vi "Test Beep.vi"() -> ()   [LabVIEW 2016, in "CS++BeepActor.lvlib"]
doc: "Test Beep.vi"
uses:
  CS++BeepActor.lvlib
  Beep.lvclass
panel:
  in  "Duration":dbl[unit]=0.1
  in  "Frequency (440)":dbl[unit]=440.0
  in  "Use System Alert?":bool
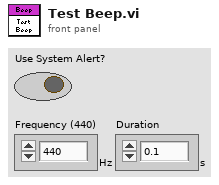
[diagram p1: front panel]
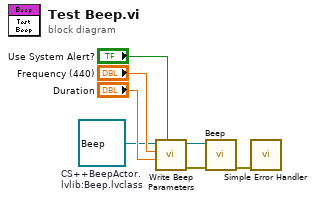
[diagram p0: block diagram]
diagram:
  w1 = refnum<class "Beep.lvclass"> refnum  # CS++BeepActor.lvlib:Beep.lvclass
  n1 = call "Write Beep Parameters.vi"("Use System Alert?"="Use System Alert?", "Duration"="Duration", "Frequency (440)"="Frequency (440)", "Beep in"=w1) -> ("error out"=w2:errorcluster, "Beep out"=w3:refnum<class "Beep.lvclass">)  [unwired: 6 in]
  n2 = call "Beep.vi"("error in (no error)"=w2, "Beep in"=w3) -> ("error out"=w4:errorcluster)  [unwired: 8 in, 1 out]
  n3 = call <vilib>:"Simple Error Handler.vi"("error in (no error)"=w4) -> ()  [unwired: 4 in, 5 out]
